vi "Post Process Photon Counting.vi"(0 "pInputImage":i32, 1 "iNumframes":i32, 2 "pfThreshold":sgl, 3 "iWidth":i32, 5 "pOutputImage":i32, 7 "iOutputBufferSize":i32, 9 "iNumImages":i32, 12 "iNumberOfThresholds":i32, 13 "iHeight":i32) -> (4 "pInputImage out":i32, 6 "pOutputImage out":i32, 8 "pfThreshold out":sgl, 10 "function return":u32)   [LabVIEW 2018, in "AndorSDK.lvlib"]
doc: "EXPNETTYPE unsigned int WINAPI PostProcessPhotonCounting(at_32 * pInputImage, at_32 * pOutputImage, int iOutputBufferSize, int iNumImages, int iNumframes, int iNumberOfThresholds, float * pfThreshold, int iHeight, int iWidth);"
uses:
  AndorSDK.lvlib
  ATMCD32D.dll
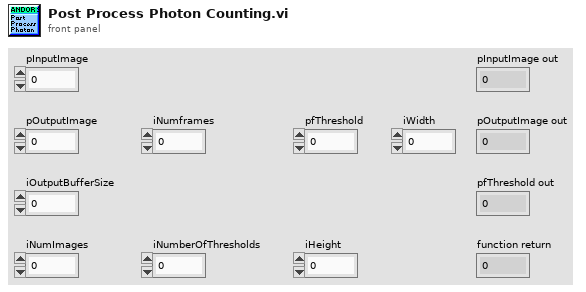
[diagram p1: front panel]
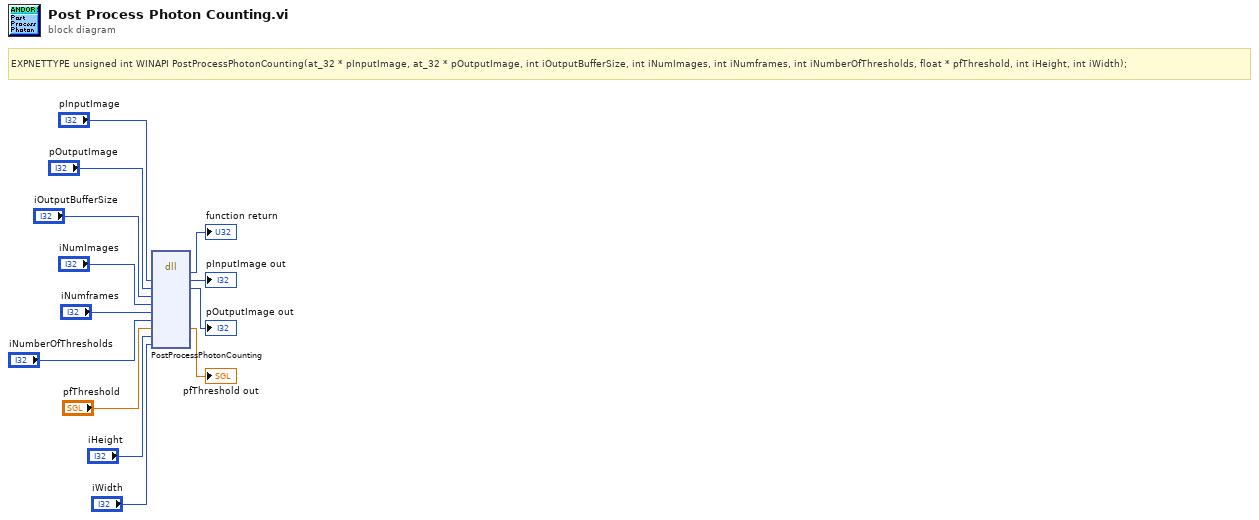
[diagram p0: block diagram]
diagram:
  # "EXPNETTYPE unsigned int WINAPI PostProcessPhotonCounting(at_32 * pInputImage, at_32 * pOutputImage, int iOutputBufferSize, int iNumImages, int iNumframes, int iNumberOfThresholds, float * pfThreshold, int iHeight, int iWidth);"
  n1 = dll-call lib="PTH2babs E\nPersönliches02 - Arbeit03-HiwijobsLabviewCodelibANDOR\tAndor SDK\nATMCD32D.*" fn="PostProcessPhotonCounting"("pInputImage"="pInputImage", "pOutputImage"="pOutputImage", "iOutputBufferSize"="iOutputBufferSize", "iNumImages"="iNumImages", "iNumframes"="iNumframes", "iNumberOfThresholds"="iNumberOfThresholds", "pfThreshold"="pfThreshold", "iHeight"="iHeight", "iWidth"="iWidth") -> (→"function return":u32, "pInputImage"=→"pInputImage out":i32, "pOutputImage"=→"pOutputImage out":i32, "pfThreshold"=→"pfThreshold out":sgl)  [unwired: 9 in, 2 out]
